vi "CATLabEnv Main.vi"() -> ()   [LabVIEW 2017]
doc: "Use this template to build a producer/consumer design pattern with events to produce queue items. Use this design pattern instead of the User Interface Event Handler pattern for user interfaces when you want to execute code asynchronously in response to an event without slowing the user interface responsiveness."
uses:
  controls/stateMachine.ctl
panel:
  out "error out":errorcluster
  in  "stop":bool
  in  "Enqueue Element":bool
  in  "shutdown":bool
  in  "Tab Control":enum32{"SCADA", "Setup", "Parameters"}(tab)
  out "chart_probe4":dbl(graph)
  out "chart_probe2":dbl(graph)
  out "chart_probe3":dbl(graph)
  out "chart_probe1":dbl(graph)
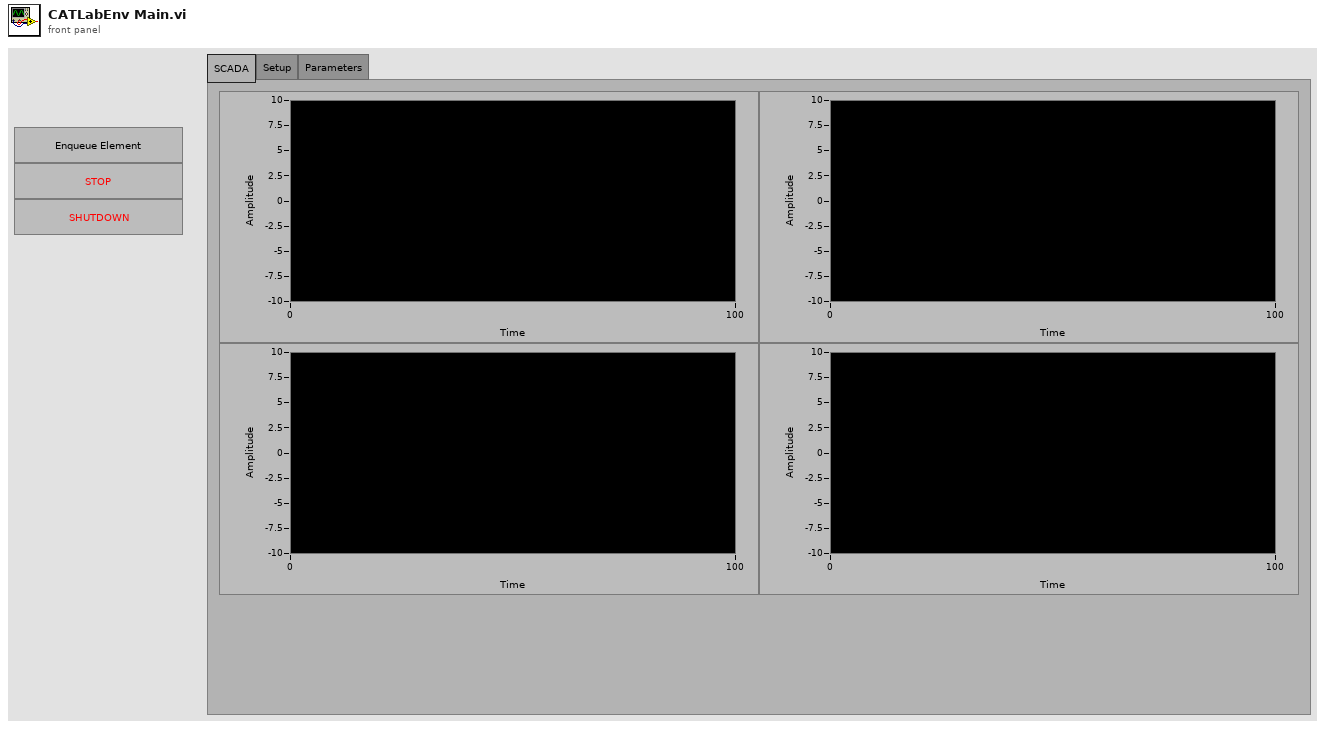
[diagram p1: front panel]
types:
  T1 = typedef "stateMachine.ctl" = enum16{"Initialize", "Start", "Pause", "Stop", "Shutdown"}
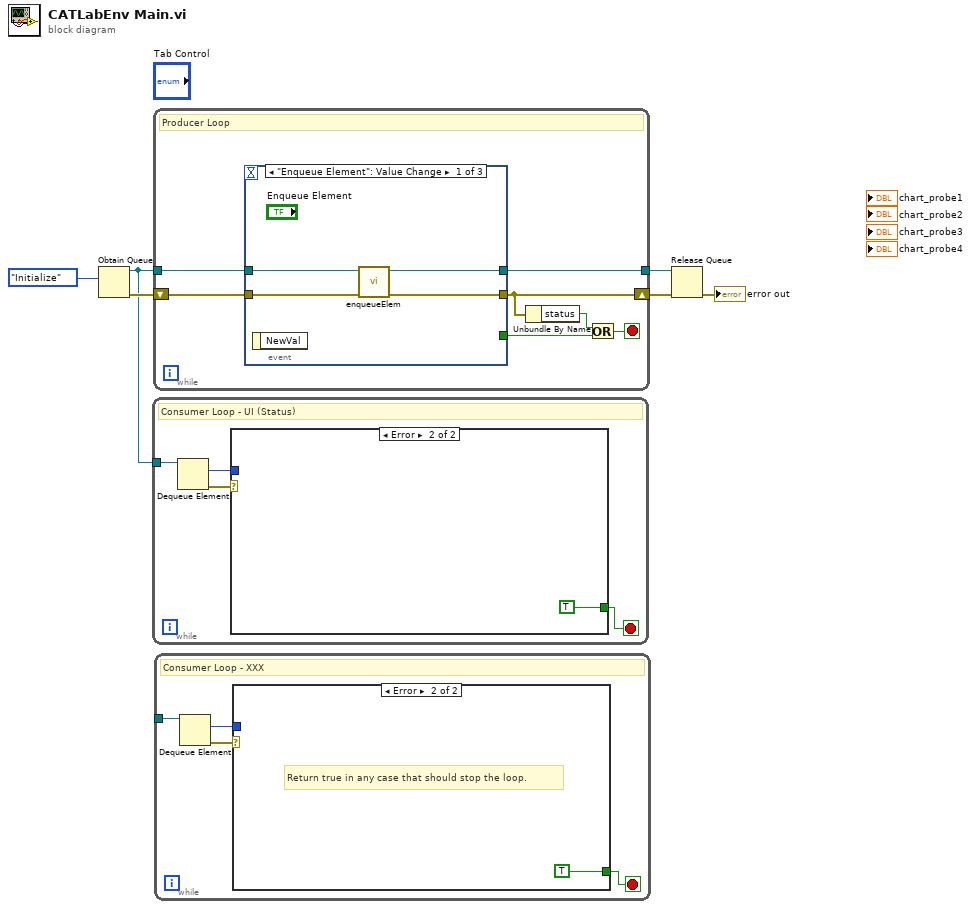
[diagram p0: block diagram]
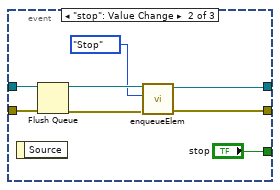
[diagram p4: hidden frame]
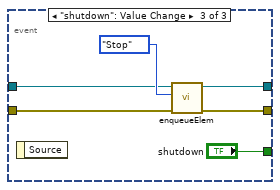
[diagram p5: hidden frame]
diagram:
  n1 = Obtain Queue(element data type=stateMachine."Initialize") -> (queue out=w4:refnum<queue>, error out=w6:errorcluster)  [unwired: 4 in, 1 out]
  n2 = while {
    tunnel: w4 -> [w10]
    stop <- w7 stop-if-true
    # "Consumer Loop - UI (Status)"
    n3 = Dequeue Element(queue=w10) -> (element=w8:T1, error out=w9:errorcluster)  [unwired: 2 in, 2 out]
    n4 = case shown="Error" w9 {
      tunnel: w8 -> [_ _]
      tunnel: [_ TRUE] -> w7
      frame No Error {
        # "Process the data here."
      }
      frame Error {
      }
    }
  }
  n5 = while {
    shift-right: [w14] -> w5
    shift-left: w6 -> [w17]
    tunnel: w4 -> [w18]
    tunnel: [w12] -> w2
    stop <- w15 stop-if-true
    # "Producer Loop"
    n6 = event shown="[0] \"Enqueue Element\": Value Change" {
      selector: _ -> [_ _ _]
      dyn-events: _ -> [_ _ _]
      timeout: _ -> [_ _ _]
      tunnel: w18 -> [w20 w28 w32]
      tunnel: w17 -> [w21 w29 w34]
      tunnel: [w22 w27 w33] -> w14
      tunnel: [_ "stop" "shutdown"] -> w16
      tunnel: [w19 w23 w31] -> w12
      event "Enqueue Element": Value Change {
        n7 = event-data() -> ()  [unwired: 1 in, 1 out]
        n8 = call "enqueueElem.vi"("error_in"=w21, "queue_in"=w20) -> ("error_out"=w22:errorcluster, "queue_out"=w19:refnum<queue>)  [unwired: 8 in]
      }
      event "stop": Value Change {
        n9 = event-data() -> ()  [unwired: 1 in, 1 out]
        n10 = Flush Queue(queue=w28, error in (no error)=w29) -> (queue out=w25:refnum<queue>, error out=w26:errorcluster)  [unwired: 1 out]
        n11 = call "enqueueElem.vi"("error_in"=w26, "element"=stateMachine."Stop", "queue_in"=w25) -> ("error_out"=w27:errorcluster, "queue_out"=w23:refnum<queue>)  [unwired: 7 in]
      }
      event "shutdown": Value Change {
        n12 = event-data() -> ()  [unwired: 1 in, 1 out]
        n13 = call "enqueueElem.vi"("error_in"=w34, "element"=stateMachine."Stop", "queue_in"=w32) -> ("error_out"=w33:errorcluster, "queue_out"=w31:refnum<queue>)  [unwired: 7 in]
      }
    }
    n14 = Unbundle By Name(w14) -> ("status"=w13:bool)
    n15 = Or(x=w13, y=w16) -> (x .or. y?=w15:bool)
  }
  n16 = while {
    tunnel: _ -> [w40]
    stop <- w37 stop-if-true
    # "Consumer Loop - XXX"
    n17 = Dequeue Element(queue=w40) -> (element=w38:T1, error out=w39:errorcluster)  [unwired: 2 in, 2 out]
    n18 = case shown="Error" w39 {
      tunnel: w38 -> [_ _]
      tunnel: [_ TRUE] -> w37
      frame No Error {
        # "Process the data here."
      }
      frame Error {
        # "Return true in any case that should stop the loop."
      }
    }
  }
  n19 = Release Queue(queue=w2, error in (no error)=w5) -> (error out=→"error out":errorcluster)  [unwired: 1 in, 2 out]
